vi "Application_viRefRegistration.vi"(1 "VI Refnum":refnum<vi>, 2 "Name (VI Name when empty)":string, 3 "Command":T2(ring), 5 "error in (no error)":errorcluster, 9 "Skip":bool) -> (17 "List":T1(array[cluster]), 19 "error out":errorcluster)   [LabVIEW 2016]
doc: "Tabelle in welche VIReferenzen mit Namen und Zeitstempel gespeichert und entfernt werden können. Z.B. zum erfassen von dynamischen Ref.-Objekten\n\n25.04.14 / sige"
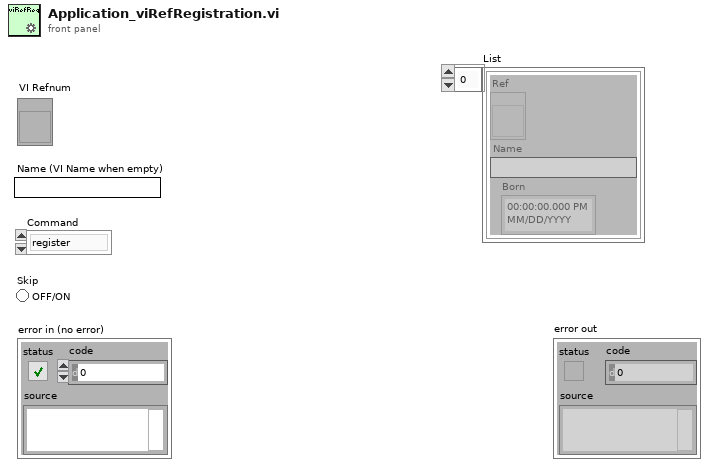
[diagram p1: front panel]
types:
  T1 = cluster{"Ref":refnum<vi>, "Name":string, "Born":timestamp}[]
  T2 = enum16{"register", "unregister", "getList", "clearList"}
  T3 = cluster{"Ref":refnum<vi>, "Name":string, "Born":timestamp}
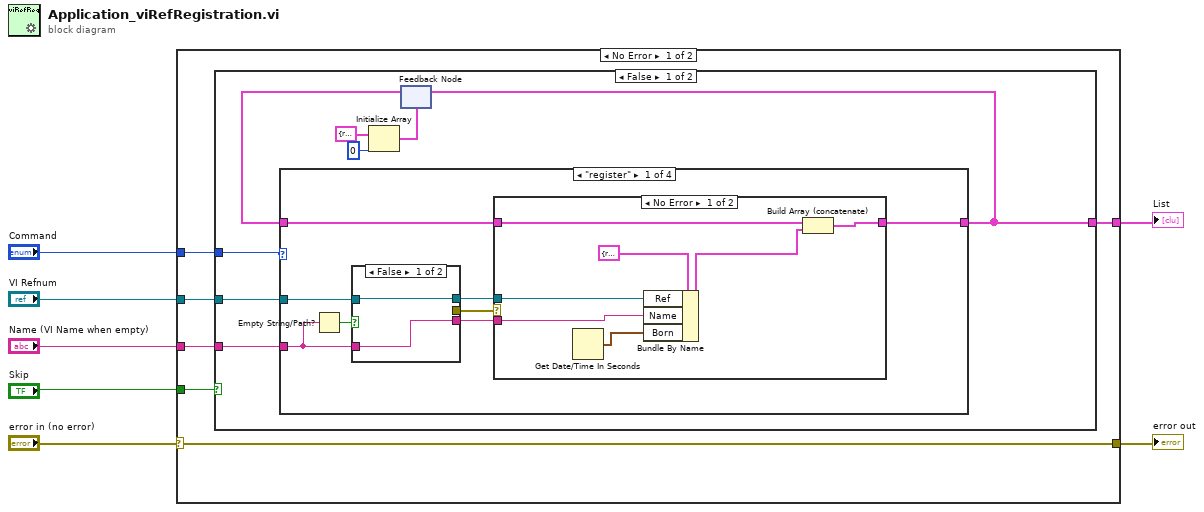
[diagram p0: block diagram]
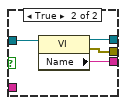
[diagram p2: hidden frame]
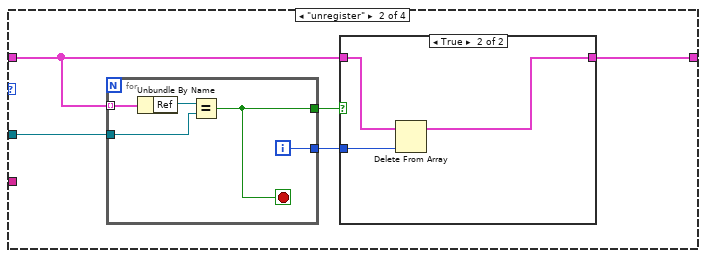
[diagram p4: hidden frame]
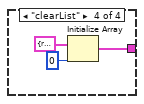
[diagram p7: hidden frame]
diagram:
  n1 = case shown="No Error" "error in (no error)" {
    selector: "error in (no error)" -> [w13 w62]
    tunnel: [w13 w62] -> w6
    tunnel: "VI Refnum" -> [w11 _]
    tunnel: "Command" -> [w12 _]
    tunnel: [w10 _] -> w3
    tunnel: "Skip" -> [w9 _]
    tunnel: "Name (VI Name when empty)" -> [w8 _]
    frame No Error {
      n2 = case shown="False" w9 {
        tunnel: w12 -> [w21 _]
        tunnel: w11 -> [w16 _]
        tunnel: [w15 _] -> w10
        tunnel: w8 -> [w14 _]
        frame False {
          n3 = Initialize Array(T3 {"Ref"=refnum, "Name"="", "Born"=timestamp(0 s since 1904-01-01)}, 0 ("dimension size")) -> (w18:T1)
          n4 = feedback #1(w18) -> (w17:T1)
          n5 = case shown="\"register\"" w21 {
            tunnel: [w29 w45 w58 w59] -> w15
            tunnel: w17 -> [w25 w47 w58 _]
            tunnel: w16 -> [w28 w48 _ _]
            tunnel: w14 -> [w22 _ _ _]
            frame "register" {
              n6 = Empty String/Path?(string/path=w22) -> (empty?=w23:bool)
              n7 = case shown="False" w23 {
                tunnel: w28 -> [w30 w35]
                tunnel: [w30 w34] -> w27
                tunnel: [w31 w33] -> w26
                tunnel: [_ w32] -> w24
                tunnel: w22 -> [w31 _]
                frame False {
                }
                frame True {
                  n8 = property class="VI"(reference=w35) -> (reference out=w34:refnum<vi>, error out=w32:errorcluster, "Name"=w33:string)  [unwired: 1 in]
                }
              }
              n9 = case shown="No Error" w24 {
                tunnel: [w41 w43] -> w29
                tunnel: w27 -> [w39 _]
                tunnel: w26 -> [w38 _]
                tunnel: w25 -> [w36 w43]
                frame No Error {
                  n10 = Get Date/Time In Seconds() -> (seconds since 1Jan1904=w37:timestamp)
                  n11 = Bundle By Name(cluster=T3 {"Ref"=refnum, "Name"="", "Born"=timestamp(0 s since 1904-01-01)}, "Ref"=w39, "Name"=w38, "Born"=w37) -> (w40:T3)
                  n12 = Build Array (concatenate)(w36, w40) -> (w41:T1)
                }
                frame Error {
                }
              }
            }
            frame "unregister" {
              n13 = for {
                tunnel: w47 -> [w57] mode=indexing
                tunnel: w48 -> [w55]
                tunnel: [w54] -> w46
                tunnel: [w53] -> w44
                i -> [w53]
                stop <- w54 stop-if-true
                n14 = Unbundle By Name(w57) -> ("Ref"=w56:refnum<vi>)
                n15 = Equal?(x=w56, y=w55) -> (x = y?=w54:bool)
              }
              n16 = case shown="True" w46 {
                tunnel: w47 -> [w49 w51]
                tunnel: [w49 w50] -> w45
                tunnel: w44 -> [_ w52]
                frame False {
                }
                frame True {
                  n17 = Delete From Array(array=w51, index=w52) -> (array with subset deleted=w50:T1)  [unwired: 1 in, 1 out]
                }
              }
            }
            frame "getList", Default {
            }
            frame "clearList" {
              n18 = Initialize Array(T3 {"Ref"=refnum, "Name"="", "Born"=timestamp(0 s since 1904-01-01)}, 0 ("dimension size")) -> (w59:T1)
            }
          }
          n19 = feedback-in #1(w15) -> ()
        }
        frame True {
        }
      }
    }
    frame Error {
    }
  }
  "error out" <- w6
  "List" <- w3
